vi "Configure PA TIME TEST.vi"(8 "error in (no error)":errorcluster, 9 "Pause time":dbl min=0.0 max=999.0 step=0.1 format="%.1f", 10 "Step":T1=1 min=1 max=99 step=1, 11 "VISA resource in":refnum<visa-resource-name>) -> (0 "error out":errorcluster, 3 "VISA resource out":refnum<visa-resource-name>)   [LabVIEW 2025, in "Chroma 19052.lvlib"]
uses:
  <instrlib>/Chroma 19052/Chroma 19052.lvlib
  <instrlib>/Chroma 19052/Public/Utility/Type Def/steps--numeric.ctl
panel:
  # "Set PA TIME"
  # "0 = CONT.\n0.3 <= time <= 999.0"
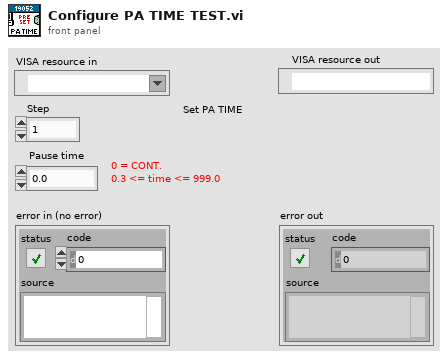
[diagram p1: front panel]
types:
  T1 = typedef "Chroma 19052.lvlib/steps--numeric.ctl" = u8
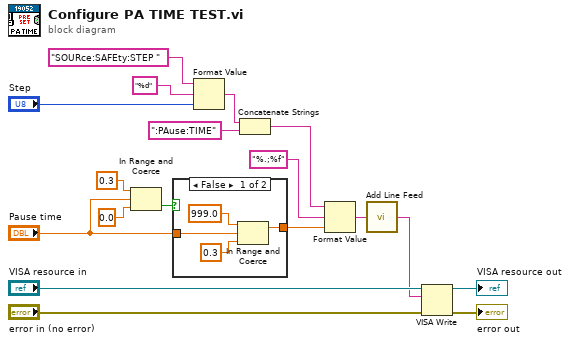
[diagram p0: block diagram]
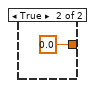
[diagram p2: hidden frame]
diagram:
  n1 = In Range and Coerce(upper limit=0.3, x="Pause time", lower limit=0.0) -> (In Range?=w2:bool)  [unwired: 1 out]
  n2 = case shown="False" w2 {
    tunnel: "Pause time" -> [w20 _]
    tunnel: [w19 0.0] -> w10
    frame False {
      n3 = In Range and Coerce(upper limit=999.0, x=w20, lower limit=0.3 ("upper limit")) -> (coerced(x)=w19:dbl)  [unwired: 1 out]
    }
    frame True {
    }
  }
  n4 = Format Value(string ("")="SOURce:SAFEty:STEP ", format string="%d", value (0)="Step") -> (output string=w12:string)
  n5 = Concatenate Strings(w12, ":PAuse:TIME") -> (w9:string)
  n6 = Format Value(string ("")=w9, format string="%.;%f", value (0)=w10) -> (output string=w7:string)
  n7 = call <instrlib>:"Add Line Feed.vi"("Command string"=w7) -> ("Concatenated string"=w6:string)  [unwired: 4 in]
  n8 = VISA Write(VISA resource name="VISA resource in", write buffer=w6, error in (no error)="error in (no error)") -> (VISA resource name out=→"VISA resource out":refnum<visa-resource-name>, error out=→"error out":errorcluster)  [unwired: 1 out]
